vi "SetRoutingKey.vi"(9 "SendTo":string, 10 "MessageClassType":T1, 11 "Message Header in":T2) -> (3 "Message Header out":T2)   [LabVIEW 2017]
uses:
  <vilib>/addons/InsightCM/MessageBus/Base/controls/MessageHeader.ctl
  <vilib>/addons/InsightCM/MessageBus/Base/controls/KeyValuePair.ctl
  <vilib>/addons/InsightCM/MessageBus/Base/controls/MessageClassType.ctl
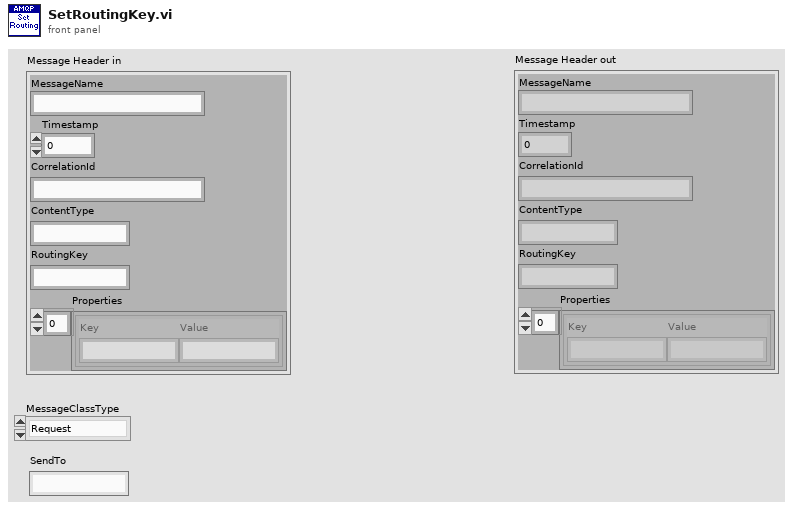
[diagram p1: front panel]
types:
  T1 = typedef "MessageClassType.ctl" = enum16{"Request", "Response", "Broadcast", "RoutedMessage"}
  T2 = typedef "MessageHeader.ctl" = cluster{"MessageName":string, "Timestamp":i64, "CorrelationId":string, "ContentType":string, "RoutingKey":string, "Properties":T3[]}
  T3 = typedef "KeyValuePair.ctl" = cluster{"Key":string, "Value":string}
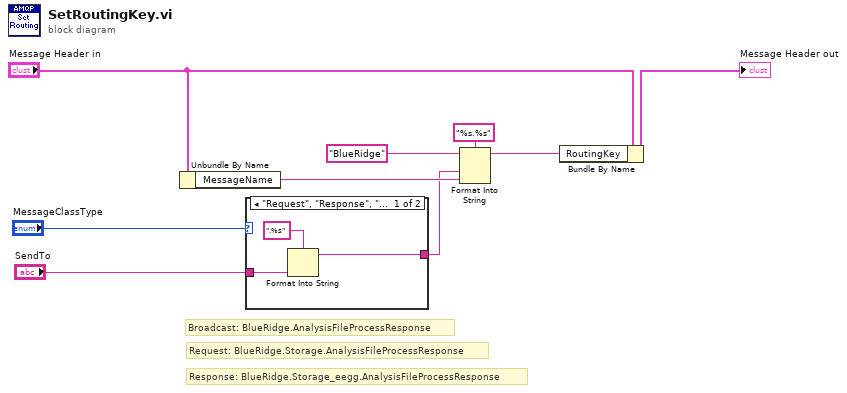
[diagram p0: block diagram]
diagram:
  # "Broadcast: BlueRidge.AnalysisFileProcessResponse"
  # "Response: BlueRidge.Storage_eegg.AnalysisFileProcessResponse"
  # "Request: BlueRidge.Storage.AnalysisFileProcessResponse"
  n1 = Unbundle By Name("Message Header in") -> ("MessageName"=w5:string)
  n2 = case shown="\"Request\", \"Response\", \"RoutedMessage\"" "MessageClassType" {
    tunnel: "SendTo" -> [w11 _]
    tunnel: [w10 _] -> w2
    frame "Request", "Response", "RoutedMessage" {
      n3 = Format Into String(format string=".%s", w11) -> (resulting string=w10:string)  [unwired: 2 in, 1 out]
    }
    frame "Broadcast" {
    }
  }
  n4 = Format Into String(format string="%s.%s", initial string="BlueRidge", w2, w5) -> (resulting string=w1:string)  [unwired: 1 in, 1 out]
  n5 = Bundle By Name(cluster="Message Header in", "RoutingKey"=w1) -> (→"Message Header out":T2)
